vi "Read Waveform (Multiple).vi"(6 "Timeout (10000 ms)":i32=10000 min=1, 8 "error in (no error)":errorcluster, 10 "Trace (0: U1)":i32[](array[ring]) items=["U1", "I1", "U2", "I2", "U3", "I3", "U4", "I4", "U5", "I5", "U6", "I6", "Speed", "Torque", "AUX1", "AUX2"], 11 "VISA resource name":refnum<visa-resource-name>) -> (0 "error out":errorcluster, 2 "Waveform Data":T1(graph), 3 "VISA resource name out":refnum<visa-resource-name>)   [LabVIEW 2021, in "Yokogawa WT1800 Series.lvlib"]
doc: "The VI waits for the acquisition to complete and returns the waveform for the trace you specified. If the instruments did not complete the acquisition within the time period you specify with the Timeout parameter, the VI returns a time out error. A common cause for a timeout error is the acquisition was not triggered. For example, the trigger level is out of range of the waveform."
uses:
  <instrlib>/Yokogawa WT1800 Series/Yokogawa WT1800 Series.lvlib
panel:
  # "ms"
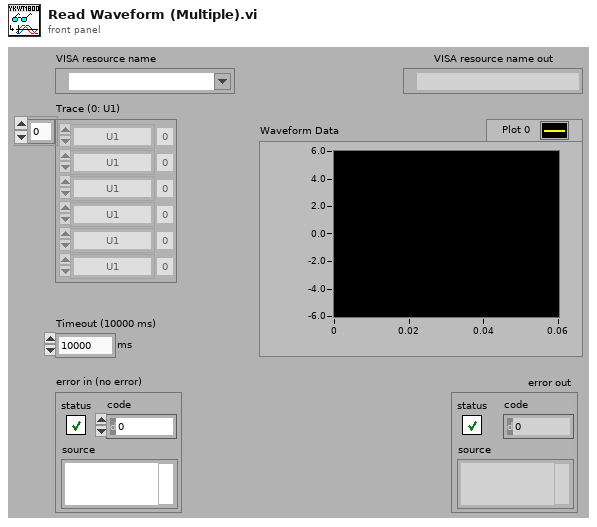
[diagram p1: front panel]
types:
  T1 = cluster{"start":dbl, "Sampling Time":dbl, "Output":dbl[]}[]
  T2 = cluster{"start":dbl, "Sampling Time":dbl, "Output":dbl[]}
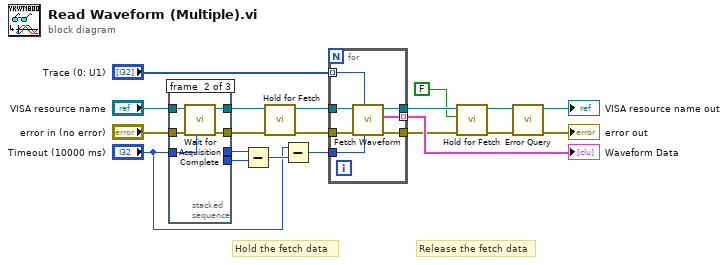
[diagram p0: block diagram]
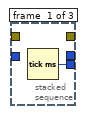
[diagram p2: hidden frame]
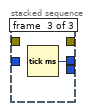
[diagram p3: hidden frame]
diagram:
  # "Release the fetch data"
  # "Hold the fetch data"
  n1 = stacked-sequence {
    tunnel: "VISA resource name" -> [_ w24 _]
    tunnel: [_ w23 _] -> w9
    tunnel: "error in (no error)" -> [_ w25 _]
    tunnel: [_ w22 _] -> w7
    tunnel: [w21 _ _] -> w15
    tunnel: "Timeout (10000 ms)" -> [_ w26 _]
    tunnel: [_ _ w27] -> w16
    frame #0 {
      n2 = Tick Count (ms)() -> (millisecond timer value=w21:u32)
    }
    frame #1 {
      n3 = call <instrlib>:"Wait for Acquisition Complete.vi"("Timeout (10000 ms)"=w26, "error in (no error)"=w25, "VISA resource name"=w24) -> ("error out"=w22:errorcluster, "VISA resource name out"=w23:refnum<visa-resource-name>)  [unwired: 7 in]
    }
    frame #2 {
      n4 = Tick Count (ms)() -> (millisecond timer value=w27:u32)
    }
  }
  n5 = Subtract(x=w16, y=w15) -> (x-y=w14:u32)
  n6 = call <instrlib>:"Hold for Fetch.vi"("error in (no error)"=w7, "VISA resource name"=w9) -> ("error out"=w6:errorcluster, "VISA resource name out"=w8:refnum<visa-resource-name>)  [unwired: 8 in]
  n7 = Subtract(x="Timeout (10000 ms)", y=w14) -> (x-y=w10:u32)
  n8 = for {
    tunnel: w10 -> [w34]
    tunnel: w6 -> [w33]
    tunnel: w8 -> [w32]
    tunnel: [w31] -> w3
    tunnel: [w30] -> w2
    tunnel: [w29] -> w18 mode=indexing
    tunnel: "Trace (0: U1)" -> [w28] mode=indexing
    n9 = call <instrlib>:"Fetch Waveform.vi"("Timeout (10000 ms)"=w34, "Trace (0: U1)"=w28, "error in (no error)"=w33, "VISA resource name"=w32) -> ("error out"=w30:errorcluster, "Waveform Data"=w29:T2, "VISA resource name out"=w31:refnum<visa-resource-name>)  [unwired: 5 in]
  }
  "Waveform Data" <- w18
  n10 = call <instrlib>:"Hold for Fetch.vi"("error in (no error)"=w2, "Hold for Fetch (T: Enable)"=FALSE, "VISA resource name"=w3) -> ("error out"=w4:errorcluster, "VISA resource name out"=w5:refnum<visa-resource-name>)  [unwired: 7 in]
  n11 = call <instrlib>:"Error Query.vi"("error in (no error)"=w4, "VISA resource name"=w5) -> ("error out"=→"error out":errorcluster, "VISA resource name out"=→"VISA resource name out":refnum<visa-resource-name>)  [unwired: 6 in, 2 out]
